vi "DeleteTone.vi"(1 "Tone Index":u16(ring) items=["Tone 1", "Tone 2", "Tone 3", "Tone 4", "Tone 5", "Tone 6", "Tone 7", "Tone 8", "Tone 9", "Tone 10"], 3 "error in (no error)":errorcluster, 4 "Selection":u16(ring)=1 items=["All Tones", "Specific Tone"], 5 "VISA resource name":refnum<visa-resource-name>) -> (0 "error out":errorcluster, 2 "VISA resource name out":refnum<visa-resource-name>)   [LabVIEW 2020, in "Active Technologies AWG3000.lvlib"]
uses:
  Active Technologies AWG3000.lvlib
panel:
  in  "ParamWave Name":string
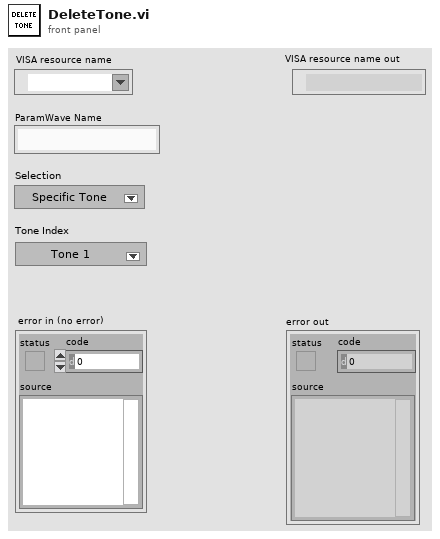
[diagram p1: front panel]
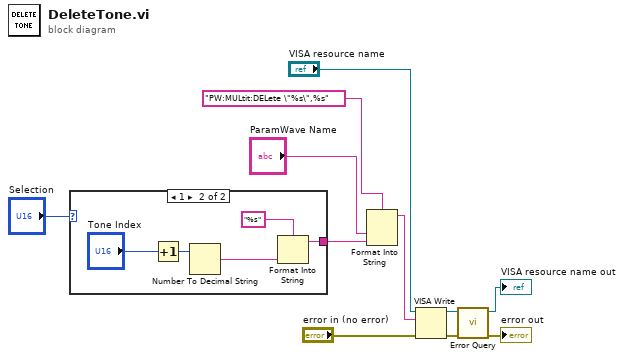
[diagram p0: block diagram]
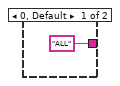
[diagram p2: hidden frame]
diagram:
  n1 = case shown="1" "Selection" {
    tunnel: ["ALL" ("write buffer") w16] -> w2
    frame 0, Default {
    }
    frame 1 {
      n2 = Increment(x="Tone Index") -> (x+1=w13:u16)
      n3 = Number To Decimal String(number=w13) -> (decimal integer string=w15:string)  [unwired: 1 in]
      n4 = Format Into String(format string="%s" ("write buffer"), w15) -> (resulting string=w16:string)  [unwired: 2 in, 1 out]
    }
  }
  n5 = Format Into String(format string="PW:MULtit:DELete \"%s\",%s" ("write buffer"), "ParamWave Name", w2) -> (resulting string=w5:string)  [unwired: 2 in, 1 out]
  n6 = VISA Write(VISA resource name="VISA resource name", write buffer=w5, error in (no error)="error in (no error)") -> (VISA resource name out=w9:refnum<visa-resource-name>, error out=w8:errorcluster)  [unwired: 1 out]
  n7 = call "Error Query.vi"("error in (no error)"=w8, "VISA resource name"=w9) -> ("error out"=→"error out":errorcluster, "VISA resource name out"=→"VISA resource name out":refnum<visa-resource-name>)  [unwired: 6 in, 2 out]
